vi "exnSpectralBlock mod exp dyn x attribs.vi"(8 "error in (no error)":errorcluster, 11 "Signals in":waveform(dbl)[](array[waveform])) -> (0 "error out":errorcluster, 3 "Signals out":waveform(dbl)[](array[waveform]))   [LabVIEW 2020]
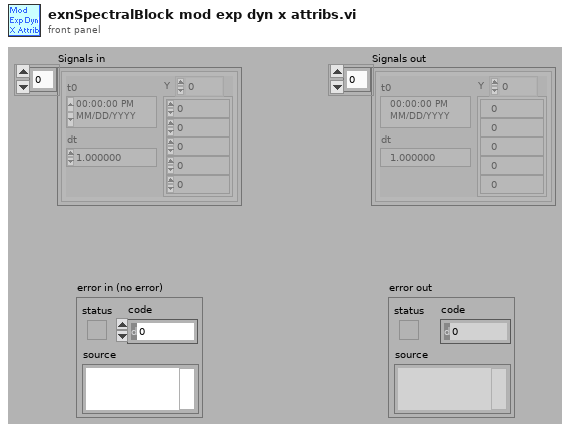
[diagram p1: front panel]
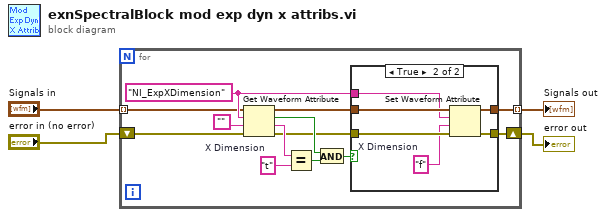
[diagram p0: block diagram]
diagram:
  n1 = for {
    tunnel: "Signals in" -> [w6] mode=indexing
    shift-right: [w17] -> w1
    shift-left: "error in (no error)" -> [w8]
    tunnel: [w16] -> w3 mode=indexing
    w12 = "t"  # X Dimension
    w15 = "NI_ExpXDimension" ("name")
    n2 = Get Waveform Attribute(4:w8, 5:"", 6:w15, 7:w6) -> (0:w7:errorcluster, 1:w14:string, 2:w9:bool, 3:w5:waveform(dbl))
    n3 = Equal?(x=w14, y=w12) -> (x = y?=w10:bool)
    n4 = And(x=w9, y=w10) -> (x .and. y?=w13:bool)
    n5 = case shown="True" w13 {
      tunnel: w5 -> [w19 w25]
      tunnel: w7 -> [w18 w24]
      tunnel: [w18 w23] -> w17
      tunnel: [w19 w22] -> w16
      tunnel: w15 -> [_ w21]
      frame False {
      }
      frame True {
        w20 = "f"  # X Dimension
        n6 = Set Waveform Attribute(4:w24, 5:w20, 6:w21, 7:w25) -> (0:w23:errorcluster, 3:w22:waveform(dbl))  [unwired: 1 out]
      }
    }
  }
  "Signals out" <- w3
  "error out" <- w1
